vi "LaunchTestMachine.vi"() -> ()   [LabVIEW 2021]
uses:
  <vilib>/ActorFramework/Message Enqueuer/Message Enqueuer.lvclass
  <vilib>/ActorFramework/Report Error Msg/Report Error Msg.lvclass/Report Error Msg.ctl
  <vilib>/ActorFramework/Message Enqueuer/Message Enqueuer.lvclass/Message Enqueuer.ctl
  AsmTestMachine/AsmTestMachine/AsmTestMachine.lvclass
  C:/Program Files (x86)/National Instruments/LabVIEW 2021/vi.lib/ActorFramework/Actor/Actor.lvclass
  Source/ActorStateMachine/ActorStateMachine Messages/ASM.Settings.ContinueEventRate Msg/ASM.Settings.ContinueEventRate Msg.lvclass/ASM.Settings.ContinueEventRate Msg.ctl
  Source/ActorStateMachine/ActorStateMachine Messages/ASM.Settings.AutoContinue Msg/ASM.Settings.AutoContinue Msg.lvclass/ASM.Settings.AutoContinue Msg.ctl
  Source/ActorStateMachine/ActorStateMachine Messages/ASM.Event.Error Msg/ASM.Event.Error Msg.lvclass/ASM.Event.Error Msg.ctl
  <vilib>/ActorFramework/Message Enqueuer/Enqueue.vi
  <vilib>/ActorFramework/Report Error Msg/Report Error Msg.lvclass
  C:/Program Files (x86)/National Instruments/LabVIEW 2021/vi.lib/ActorFramework/Message/Message.lvclass
  Source/ActorStateMachine/ActorStateMachine Messages/ASM.Settings.ContinueEventRate Msg/ASM.Settings.ContinueEventRate Msg.lvclass
  Source/ActorStateMachine/ActorStateMachine Messages/ASM.Settings.AutoContinue Msg/ASM.Settings.AutoContinue Msg.lvclass
  Source/ActorStateMachine/ActorStateMachine Messages/ASM.Event.Quit Msg/ASM.Event.Quit Msg.lvclass
  Source/ActorStateMachine/ActorStateMachine Messages/ASM.Event.Restart Msg/ASM.Event.Restart Msg.lvclass
  Source/ActorStateMachine/ActorStateMachine Messages/ASM.Event.SetUp Msg/ASM.Event.SetUp Msg.lvclass
  Source/ActorStateMachine/ActorStateMachine Messages/ASM.Event.Enable Msg/ASM.Event.Enable Msg.lvclass
  Source/ActorStateMachine/ActorStateMachine Messages/ASM.Event.Start Msg/ASM.Event.Start Msg.lvclass
  Source/ActorStateMachine/ActorStateMachine Messages/ASM.Event.Stop Msg/ASM.Event.Stop Msg.lvclass
  Source/ActorStateMachine/ActorStateMachine Messages/ASM.Event.Continue Msg/ASM.Event.Continue Msg.lvclass
  Source/ActorStateMachine/ActorStateMachine Messages/ASM.Event.Error Msg/ASM.Event.Error Msg.lvclass
  Source/ActorStateMachine/ActorStateMachine Messages/ASM.Event.Resume Msg/ASM.Event.Resume Msg.lvclass
  <vilib>/ActorFramework/Message Priority Queue/Priority Enqueue.vi
  <vilib>/ActorFramework/Actor/Actor.lvclass
panel:
  in  "ASMs":i32[](listbox)
  in  "NumContinueEventRate [ms]":u32=100 caption="Continue Event Rate [ms]"
  in  "BtnAutoContinue":bool=TRUE caption="Auto Continue"
  in  "BtnContinue":bool
  in  "BtnResume":bool
  in  "BtnError":bool
  in  "BtnQuit":bool
  in  "BtnStop":bool
  in  "BtnStart":bool
  in  "BtnEnable":bool
  in  "BtnSetUp":bool
  in  "BtnRestart":bool
  out "error out":errorcluster
  in  "BtnLaunchNewAsm":bool
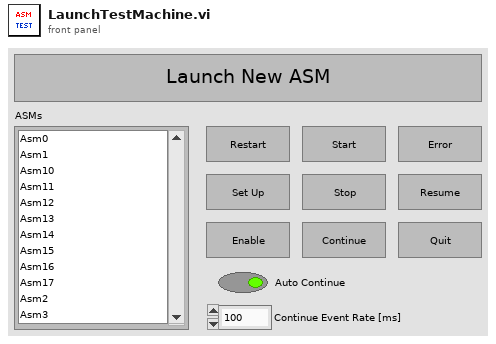
[diagram p1: front panel]
types:
  T1 = map{string, refnum<class "Message Enqueuer.lvclass">}
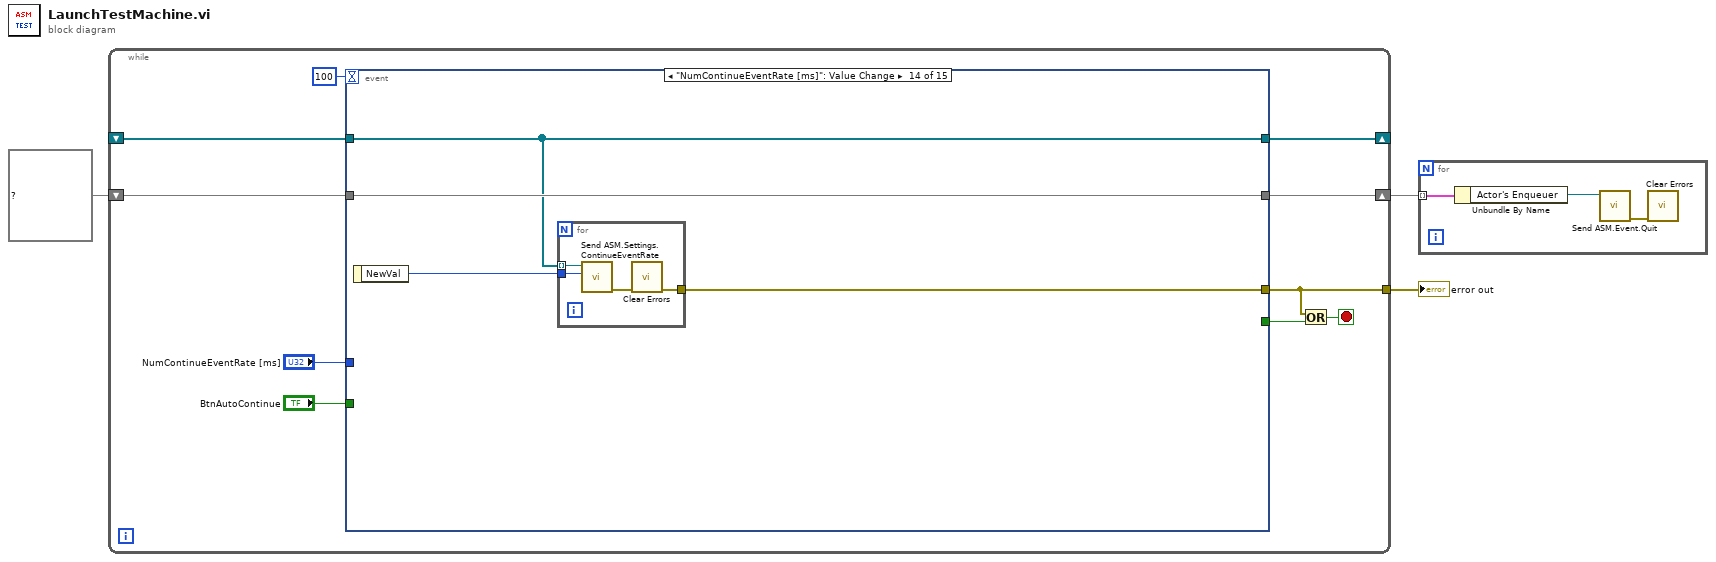
[diagram p0: block diagram]
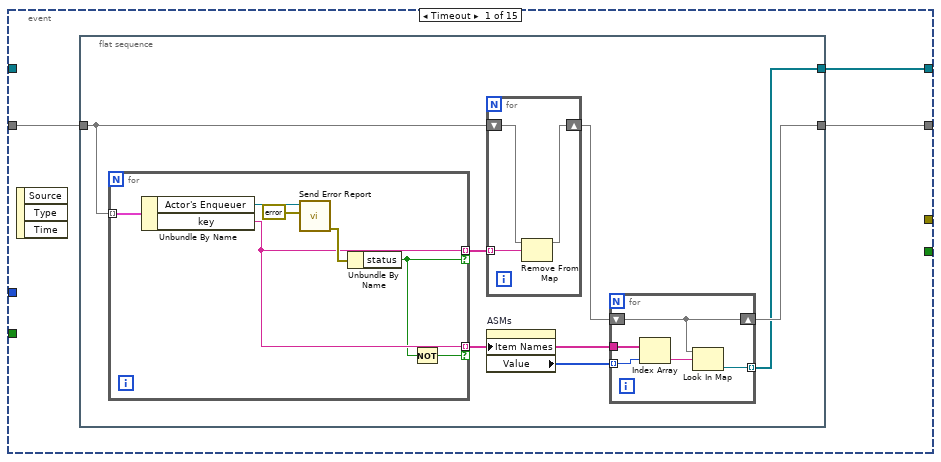
[diagram p2: hidden frame]
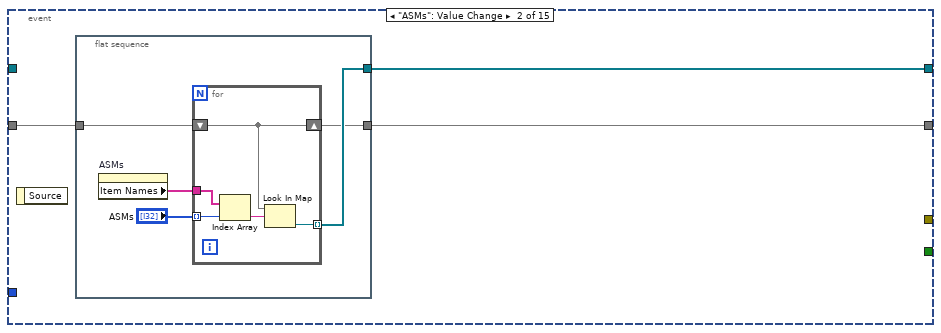
[diagram p3: hidden frame]
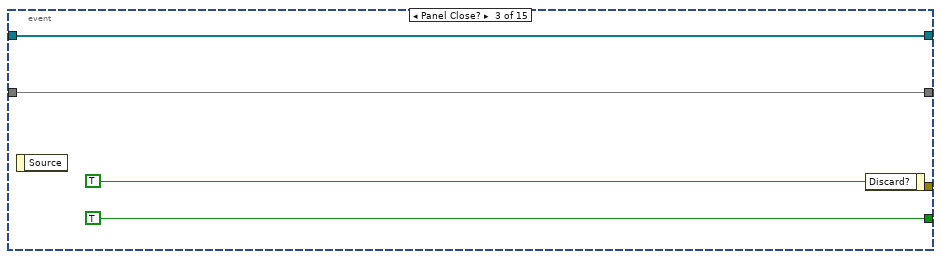
[diagram p4: hidden frame]
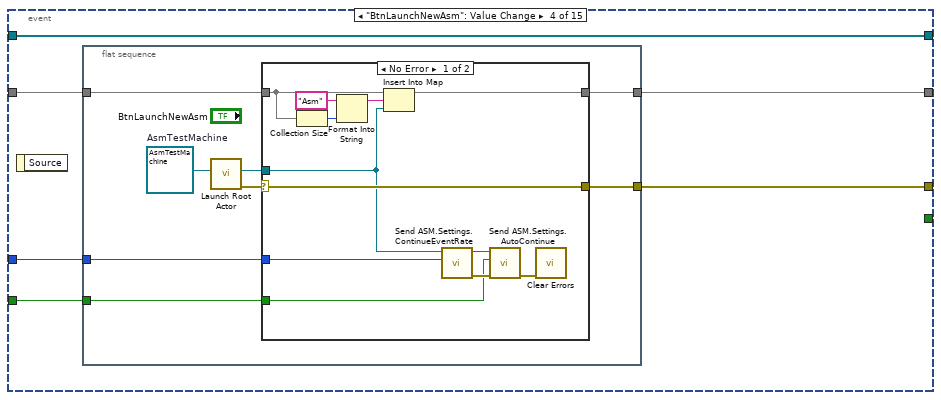
[diagram p5: hidden frame]
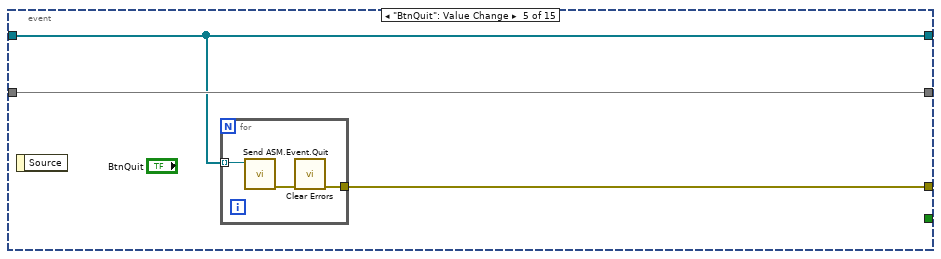
[diagram p7: hidden frame]
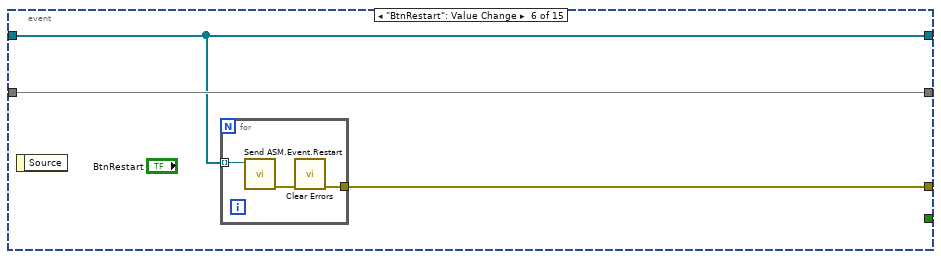
[diagram p8: hidden frame]
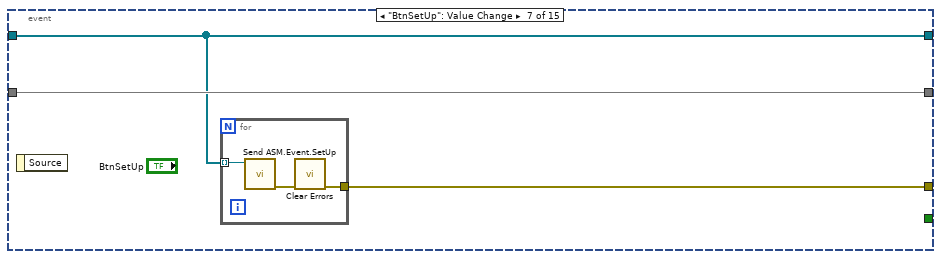
[diagram p9: hidden frame]
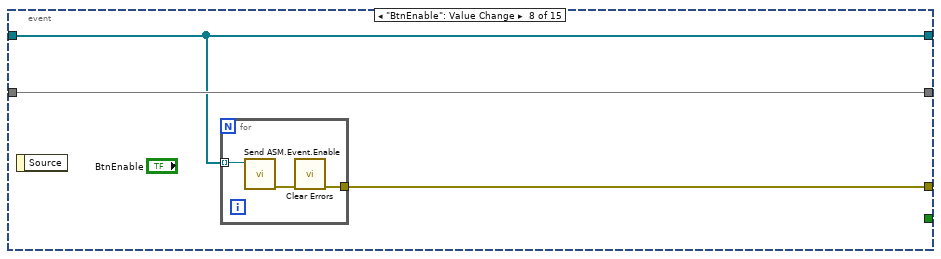
[diagram p10: hidden frame]
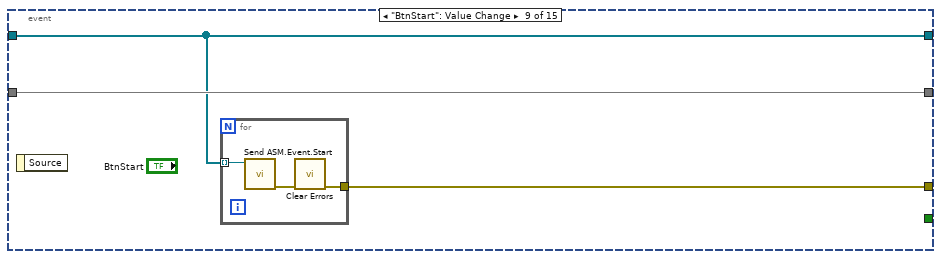
[diagram p11: hidden frame]
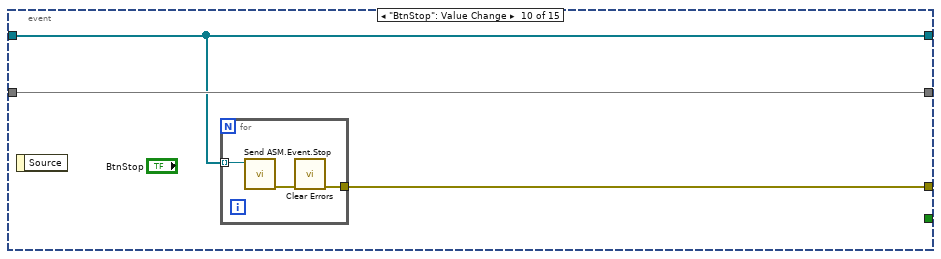
[diagram p12: hidden frame]
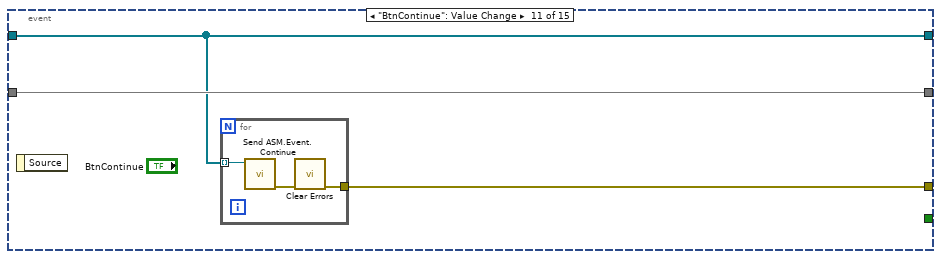
[diagram p13: hidden frame]
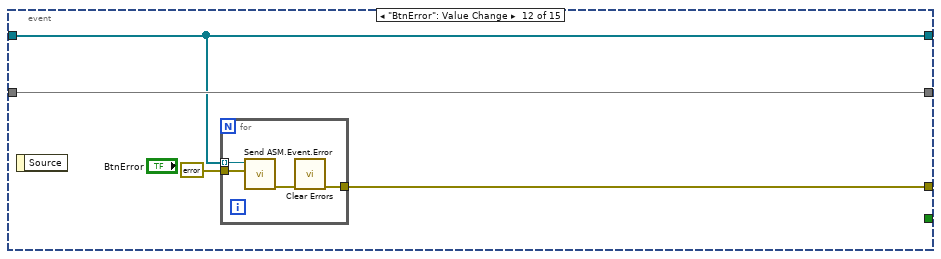
[diagram p14: hidden frame]
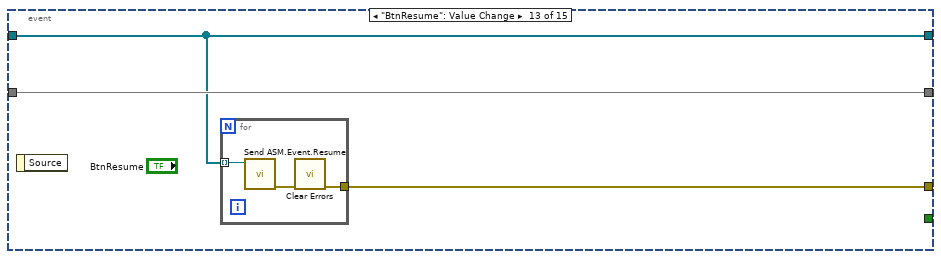
[diagram p15: hidden frame]
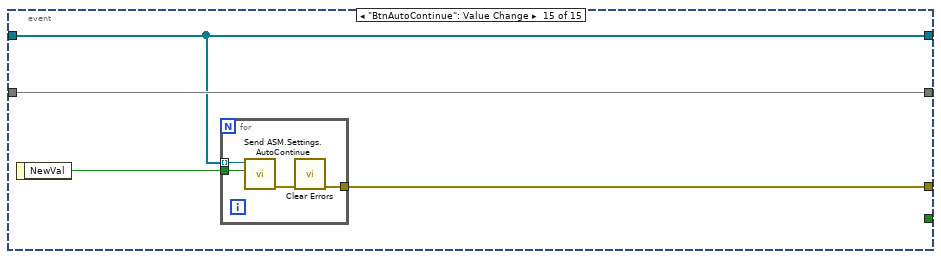
[diagram p16: hidden frame]
diagram:
  n1 = while {
    tunnel: [w13] -> w3
    shift-right: [w10] -> w1
    shift-left: T1 {} ("map") -> [w9]
    shift-right: [w7] -> _
    shift-left: _ -> [w6]
    stop <- w11 stop-if-true
    n2 = event shown="[13] \"NumContinueEventRate [ms]\": Value Change" {
      selector: _ -> [_ _ _ _ _ _ _ _ _ _ _ _ _ _ _]
      dyn-events: _ -> [_ _ _ _ _ _ _ _ _ _ _ _ _ _ _]
      timeout: 100 -> [_ _ _ _ _ _ _ _ _ _ _ _ _ _ _]
      tunnel: [_ _ TRUE _ _ _ _ _ _ _ _ _ _ _ _] -> w12
      tunnel: [_ _ _ w59 w84 w90 w97 w103 w109 w115 w121 w128 w135 w141 w149] -> w13
      tunnel: [w15 w39 w53 w61 w86 w92 w98 w104 w110 w116 w122 w129 w136 w143 w151] -> w10
      tunnel: w9 -> [w16 w41 w53 w60 w86 w92 w98 w104 w110 w116 w122 w129 w136 w143 w151]
      tunnel: [w14 w40 w52 w58 w85 w91 w96 w102 w108 w114 w120 w127 w134 w142 w150] -> w7
      tunnel: w6 -> [_ _ w52 w58 w85 w91 w96 w102 w108 w114 w120 w127 w134 w142 w150]
      tunnel: "NumContinueEventRate [ms]" -> [_ _ _ w57 _ _ _ _ _ _ _ _ _ _ _]
      tunnel: "BtnAutoContinue" -> [_ _ _ w56 _ _ _ _ _ _ _ _ _ _ _]
      event Timeout {
        n3 = event-data() -> ()  [unwired: 1 in, 3 out]
        n4 = flat-sequence {
          tunnel: w16 -> [w22]
          tunnel: [w18] -> w15
          tunnel: [w17] -> w14
          frame #0 {
            n5 = for {
              tunnel: w22 -> [w38] mode=indexing
              tunnel: [w34] -> w23 mode=indexing if=w33
              tunnel: [w34] -> w21 mode=indexing if=w32
              n6 = Unbundle By Name(w38) -> ("Actor's Enqueuer"=w37:refnum<class "Message Enqueuer.lvclass">, "key"=w34:string)
              n7 = call <vilib>:"Send Error Report.vi"("Error From Sender"=errorcluster {"status"=FALSE, "code"=0, "source"=""}, "Message Enqueuer"=w37) -> ("error out"=w35:errorcluster)  [unwired: 9 in]
              n8 = Unbundle By Name(w35) -> ("status"=w33:bool)
              n9 = Not(x=w33) -> (.not. x?=w32:bool)
            }
            n10 = for {
              tunnel: w23 -> [w31] mode=indexing
              shift-right: [w29] -> w19
              shift-left: w22 -> [w30]
              n11 = Remove From Map(10:w31, 11:w30) -> (3:w29:T1)  [unwired: 2 out]
            }
            n12 = property on="ASMs" class="LstBox (strict)"("Item Names"=w21) -> ("Value"=w20:i32[])  [unwired: 2 in, 2 out]
            n13 = for {
              tunnel: w21 -> [w28]
              tunnel: w20 -> [w27] mode=indexing
              shift-right: [w25] -> w18
              shift-left: w19 -> [w25]
              tunnel: [w24] -> w17 mode=indexing
              n14 = Index Array(array=w28, index=w27) -> (element=w26:string)
              n15 = Look In Map(map=w25, key=w26) -> (value=w24:refnum<class "Message Enqueuer.lvclass">)  [unwired: 1 in, 1 out]
            }
          }
        }
      }
      event "ASMs": Value Change {
        n16 = event-data() -> ()  [unwired: 1 in, 1 out]
        n17 = flat-sequence {
          tunnel: w41 -> [w43]
          tunnel: [w46] -> w40
          tunnel: [w42] -> w39
          frame #0 {
            n18 = property on="ASMs" class="LstBox (strict)"() -> ("Item Names"=w45:string[])  [unwired: 2 in, 2 out]
            n19 = for {
              tunnel: [w51] -> w46 mode=indexing
              tunnel: w45 -> [w50]
              tunnel: "ASMs" -> [w49] mode=indexing
              shift-right: [w47] -> w42
              shift-left: w43 -> [w47]
              n20 = Index Array(array=w50, index=w49) -> (element=w48:string)
              n21 = Look In Map(map=w47, key=w48) -> (value=w51:refnum<class "Message Enqueuer.lvclass">)  [unwired: 1 in, 1 out]
            }
          }
        }
      }
      event Panel Close? {
        n22 = event-data() -> ()  [unwired: 1 in, 1 out]
        n23 = event-data("Discard?"=TRUE) -> ()  [unwired: 1 in, 1 out]
      }
      event "BtnLaunchNewAsm": Value Change {
        n24 = event-data() -> ()  [unwired: 1 in, 1 out]
        n25 = flat-sequence {
          tunnel: [w68] -> w61
          tunnel: w60 -> [w66]
          tunnel: [w64] -> w59
          tunnel: w57 -> [w63]
          tunnel: w56 -> [w62]
          frame #0 {
            w69 = refnum<class "AsmTestMachine.lvclass"> refnum  # AsmTestMachine
            n26 = call <vilib>:"Launch Root Actor.vi"("Actor"=w69) -> ("error out"=w65:errorcluster, "Actor's Enqueuer"=w67:refnum<class "Message Enqueuer.lvclass">)  [unwired: 9 in]
            n27 = case shown="No Error" w65 {
              selector: w65 -> [w76 w83]
              tunnel: [w81 w82] -> w68
              tunnel: w67 -> [w73 _]
              tunnel: w66 -> [w80 w82]
              tunnel: [w76 w83] -> w64
              tunnel: w63 -> [w71 _]
              tunnel: w62 -> [w70 _]
              frame No Error {
                n28 = Collection Size(1:w80) -> (0:w78:i32)
                n29 = Format Into String(initial string="Asm", w78) -> (resulting string=w77:string)  [unwired: 2 in, 1 out]
                n30 = Insert Into Map(map in=w80, key=w77, value=w73) -> (map out=w81:T1)  [unwired: 2 out]
                n31 = call "Send ASM.Settings.ContinueEventRate.vi"("ContinueEventRate [ms]"=w71, "Message Enqueuer"=w73) -> ("error out"=w75:errorcluster, "Message Enqueuer out"=w74:refnum<class "Message Enqueuer.lvclass">)  [unwired: 8 in]
                n32 = call "Send ASM.Settings.AutoContinue.vi"("error in (no error)"=w75, "AutoContinue"=w70, "Message Enqueuer"=w74) -> ("error out"=w72:errorcluster)  [unwired: 7 in, 1 out]
                n33 = call <vilib>:"Clear Errors.vi"("error in (no error)"=w72) -> ()  [unwired: 5 in, 2 out]
              }
              frame Error {
              }
            }
          }
        }
      }
      event "BtnQuit": Value Change {
        n34 = event-data() -> ()  [unwired: 1 in, 1 out]
        n35 = for {
          tunnel: w85 -> [w89] mode=indexing
          tunnel: [w87] -> w84
          n36 = call "Send ASM.Event.Quit.vi"("Message Enqueuer"=w89) -> ("error out"=w88:errorcluster)  [unwired: 9 in, 1 out]
          n37 = call <vilib>:"Clear Errors.vi"("error in (no error)"=w88) -> ("error out"=w87:errorcluster)  [unwired: 5 in, 1 out]
        }
      }
      event "BtnRestart": Value Change {
        n38 = event-data() -> ()  [unwired: 1 in, 1 out]
        n39 = for {
          tunnel: w91 -> [w95] mode=indexing
          tunnel: [w93] -> w90
          n40 = call "Send ASM.Event.Restart.vi"("Message Enqueuer"=w95) -> ("error out"=w94:errorcluster)  [unwired: 9 in, 1 out]
          n41 = call <vilib>:"Clear Errors.vi"("error in (no error)"=w94) -> ("error out"=w93:errorcluster)  [unwired: 5 in, 1 out]
        }
      }
      event "BtnSetUp": Value Change {
        n42 = event-data() -> ()  [unwired: 1 in, 1 out]
        n43 = for {
          tunnel: w96 -> [w101] mode=indexing
          tunnel: [w99] -> w97
          n44 = call "Send ASM.Event.SetUp.vi"("Message Enqueuer"=w101) -> ("error out"=w100:errorcluster)  [unwired: 9 in, 1 out]
          n45 = call <vilib>:"Clear Errors.vi"("error in (no error)"=w100) -> ("error out"=w99:errorcluster)  [unwired: 5 in, 1 out]
        }
      }
      event "BtnEnable": Value Change {
        n46 = event-data() -> ()  [unwired: 1 in, 1 out]
        n47 = for {
          tunnel: w102 -> [w107] mode=indexing
          tunnel: [w105] -> w103
          n48 = call "Send ASM.Event.Enable.vi"("Message Enqueuer"=w107) -> ("error out"=w106:errorcluster)  [unwired: 9 in, 1 out]
          n49 = call <vilib>:"Clear Errors.vi"("error in (no error)"=w106) -> ("error out"=w105:errorcluster)  [unwired: 5 in, 1 out]
        }
      }
      event "BtnStart": Value Change {
        n50 = event-data() -> ()  [unwired: 1 in, 1 out]
        n51 = for {
          tunnel: w108 -> [w113] mode=indexing
          tunnel: [w111] -> w109
          n52 = call "Send ASM.Event.Start.vi"("Message Enqueuer"=w113) -> ("error out"=w112:errorcluster)  [unwired: 9 in, 1 out]
          n53 = call <vilib>:"Clear Errors.vi"("error in (no error)"=w112) -> ("error out"=w111:errorcluster)  [unwired: 5 in, 1 out]
        }
      }
      event "BtnStop": Value Change {
        n54 = event-data() -> ()  [unwired: 1 in, 1 out]
        n55 = for {
          tunnel: w114 -> [w119] mode=indexing
          tunnel: [w117] -> w115
          n56 = call "Send ASM.Event.Stop.vi"("Message Enqueuer"=w119) -> ("error out"=w118:errorcluster)  [unwired: 9 in, 1 out]
          n57 = call <vilib>:"Clear Errors.vi"("error in (no error)"=w118) -> ("error out"=w117:errorcluster)  [unwired: 5 in, 1 out]
        }
      }
      event "BtnContinue": Value Change {
        n58 = event-data() -> ()  [unwired: 1 in, 1 out]
        n59 = for {
          tunnel: w120 -> [w125] mode=indexing
          tunnel: [w123] -> w121
          n60 = call "Send ASM.Event.Continue.vi"("Message Enqueuer"=w125) -> ("error out"=w124:errorcluster)  [unwired: 9 in, 1 out]
          n61 = call <vilib>:"Clear Errors.vi"("error in (no error)"=w124) -> ("error out"=w123:errorcluster)  [unwired: 5 in, 1 out]
        }
      }
      event "BtnError": Value Change {
        n62 = event-data() -> ()  [unwired: 1 in, 1 out]
        n63 = for {
          tunnel: w127 -> [w133] mode=indexing
          tunnel: [w131] -> w128
          tunnel: errorcluster {"status"=FALSE, "code"=0, "source"=""} ("StateError") -> [w130]
          n64 = call "Send ASM.Event.Error.vi"("StateError"=w130, "Message Enqueuer"=w133) -> ("error out"=w132:errorcluster)  [unwired: 8 in, 1 out]
          n65 = call <vilib>:"Clear Errors.vi"("error in (no error)"=w132) -> ("error out"=w131:errorcluster)  [unwired: 5 in, 1 out]
        }
      }
      event "BtnResume": Value Change {
        n66 = event-data() -> ()  [unwired: 1 in, 1 out]
        n67 = for {
          tunnel: w134 -> [w139] mode=indexing
          tunnel: [w137] -> w135
          n68 = call "Send ASM.Event.Resume.vi"("Message Enqueuer"=w139) -> ("error out"=w138:errorcluster)  [unwired: 9 in, 1 out]
          n69 = call <vilib>:"Clear Errors.vi"("error in (no error)"=w138) -> ("error out"=w137:errorcluster)  [unwired: 5 in, 1 out]
        }
      }
      event "NumContinueEventRate [ms]": Value Change {
        n70 = event-data() -> ("NewVal"=w140:u32)  [unwired: 1 in]
        n71 = for {
          tunnel: w142 -> [w147] mode=indexing
          tunnel: [w145] -> w141
          tunnel: w140 -> [w144]
          n72 = call "Send ASM.Settings.ContinueEventRate.vi"("ContinueEventRate [ms]"=w144, "Message Enqueuer"=w147) -> ("error out"=w146:errorcluster)  [unwired: 8 in, 1 out]
          n73 = call <vilib>:"Clear Errors.vi"("error in (no error)"=w146) -> ("error out"=w145:errorcluster)  [unwired: 5 in, 1 out]
        }
      }
      event "BtnAutoContinue": Value Change {
        n74 = event-data() -> ("NewVal"=w148:bool)  [unwired: 1 in]
        n75 = for {
          tunnel: w150 -> [w155] mode=indexing
          tunnel: [w153] -> w149
          tunnel: w148 -> [w152]
          n76 = call "Send ASM.Settings.AutoContinue.vi"("AutoContinue"=w152, "Message Enqueuer"=w155) -> ("error out"=w154:errorcluster)  [unwired: 8 in, 1 out]
          n77 = call <vilib>:"Clear Errors.vi"("error in (no error)"=w154) -> ("error out"=w153:errorcluster)  [unwired: 5 in, 1 out]
        }
      }
    }
    n78 = Or(x=w13, y=w12) -> (x .or. y?=w11:bool)
  }
  "error out" <- w3
  n79 = for {
    tunnel: w1 -> [w158] mode=indexing
    n80 = Unbundle By Name(w158) -> ("Actor's Enqueuer"=w157:refnum<class "Message Enqueuer.lvclass">)
    n81 = call "Send ASM.Event.Quit.vi"("Message Enqueuer"=w157) -> ("error out"=w156:errorcluster)  [unwired: 9 in, 1 out]
    n82 = call <vilib>:"Clear Errors.vi"("error in (no error)"=w156) -> ()  [unwired: 5 in, 2 out]
  }
